vi "Write Command Status Ref.vi"(8 "error in (no error)":errorcluster, 10 "Command Status Ref":refnum<vi>, 11 "Command in":refnum<class "Command.lvclass">) -> (0 "error out":errorcluster, 3 "Command out":refnum<class "Command.lvclass">)   [LabVIEW 2013, in "Command Processor.lvlib" / "Command.lvlib" / "Command.lvclass"]
uses:
  Command.lvclass
  Command Status.ctl
  State Status.ctl
  Command.lvclass/Command.ctl
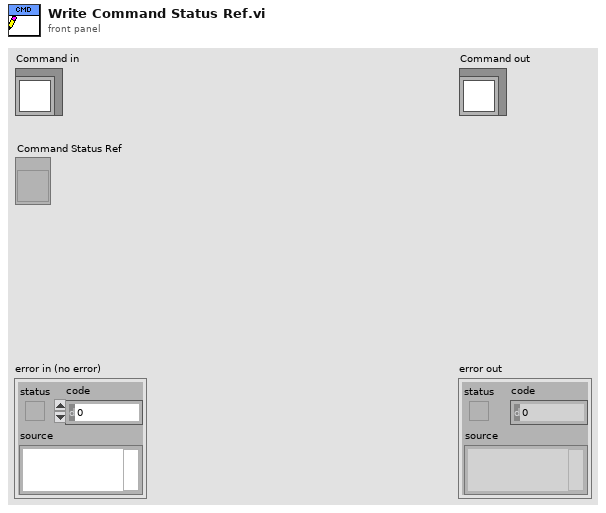
[diagram p1: front panel]
types:
  T1 = typedef "Command Processor.lvlib/Command.lvlib/Command.lvclass/Command Status.ctl" = cluster{"Command Name":string, "Current State Status":T2, "Command Start Time":timestamp, "Command End Time":timestamp, "Previous State Status":T2}
  T2 = typedef "Command Processor.lvlib/Command.lvlib/Command.lvclass/State Status.ctl" = cluster{"State Name":string, "State Entry Time":timestamp, "State Exit Time":timestamp}
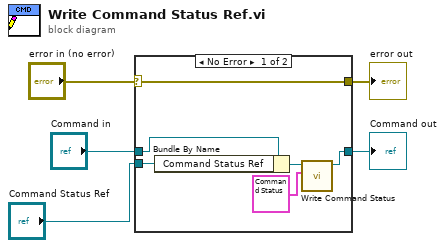
[diagram p0: block diagram]
diagram:
  n1 = case shown="No Error" "error in (no error)" {
    selector: "error in (no error)" -> [w11 w12]
    tunnel: [w11 w12] -> w4
    tunnel: [w7 w13] -> w2
    tunnel: "Command in" -> [w10 w13]
    tunnel: "Command Status Ref" -> [w9 _]
    frame No Error {
      n2 = Bundle By Name(cluster=w10, "Command Status Ref"=w9) -> (w8:refnum<class "Command.lvclass">)
      n3 = call-dynamic "Write Command Status.vi"("Command Status"=T1 {"Command Name"="Connect Command", "Current State Status"={"State Name"="", "State Entry Time"=timestamp(0 s since 1904-01-01), "State Exit Time"=timestamp(0 s since 1904-01-01)}, "Command Start Time"=timestamp(3502036417.732448 s since 1904-01-01), "Command End Time"=timestamp(0 s since 1904-01-01), "Previous State Status"={"State Name"="", "State Entry Time"=timestamp(0 s since 1904-01-01), "State Exit Time"=timestamp(0 s since 1904-01-01)}}, "Command in"=w8) -> ("Command out"=w7:refnum<class "Command.lvclass">)  [unwired: 8 in, 1 out]
    }
    frame Error {
    }
  }
  "error out" <- w4
  "Command out" <- w2
